vi "WPS_status.vi"() -> ()   [LabVIEW 2009]
panel:
  in  "Path to Exe":string="C:\\Documents and Settings\\Administrator\\My Documents\\LabViewProjects\\CTControl\\UU.W32.exe"
  out "error out":errorcluster
  out "outlet return":string
  out "Status Output":string
  in  "Password":string="WPS111rocks"
  in  "Username":string="admin"
  in  "WPS IP:Port":string="169.254.1.201:80"
  in  "Path to Batch":string="C:\\Documents and Settings\\Administrator\\My Documents\\LabViewProjects\\CTControl\\WPSrunExe.bat"
  in  "Outlet 8":bool
  in  "Outlet 7":bool
  in  "Outlet 6":bool
  in  "Outlet 5":bool
  in  "Outlet 4":bool
  in  "Outlet 3":bool
  in  "Outlet 2":bool
  in  "Outlet 1":bool
  in  "stop":bool
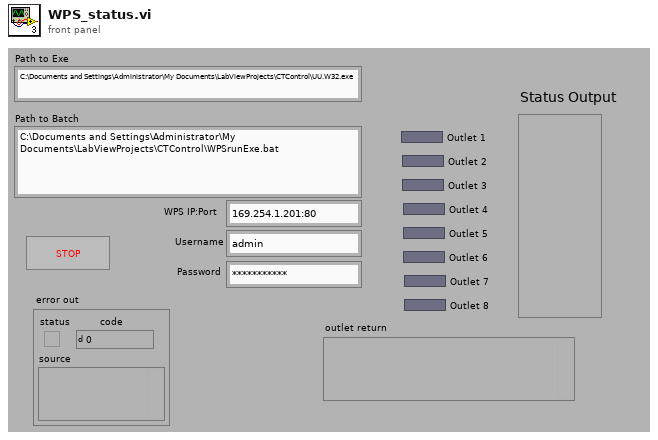
[diagram p1: front panel]
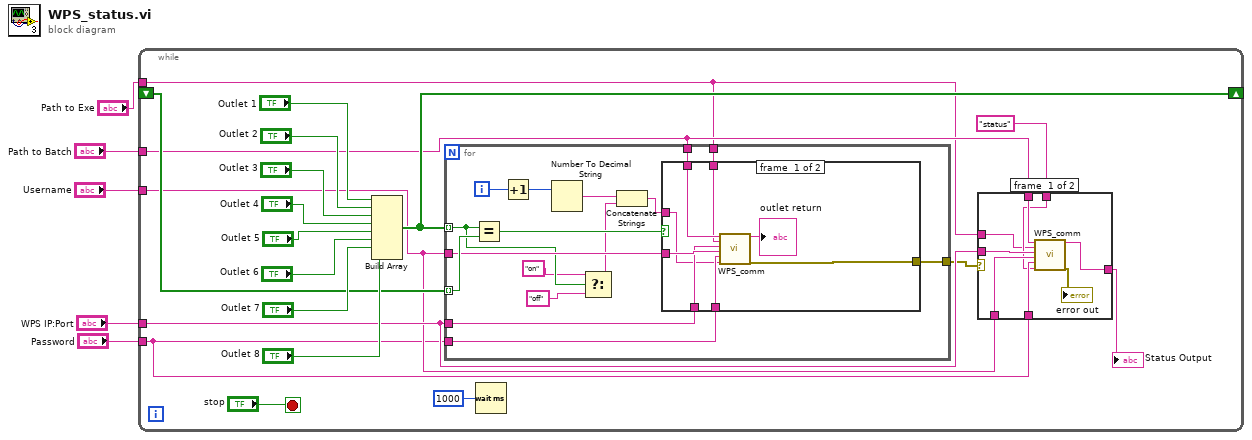
[diagram p0: block diagram]
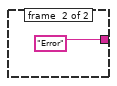
[diagram p2: hidden frame]
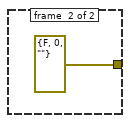
[diagram p3: hidden frame]
diagram:
  n1 = while {
    shift-right: [w16] -> _
    shift-left: _ -> [w15]
    tunnel: "Path to Batch" -> [w14]
    tunnel: "Username" -> [w12]
    tunnel: "WPS IP:Port" -> [w13]
    tunnel: "Password" -> [w11]
    tunnel: "Path to Exe" -> [w6]
    stop <- "stop" stop-if-true
    n2 = Build Array("Outlet 1", "Outlet 2", "Outlet 3", "Outlet 4", "Outlet 5", "Outlet 6", "Outlet 7", "Outlet 8") -> (w16:bool[])
    n3 = for {
      tunnel: w16 -> [w45] mode=indexing
      tunnel: w15 -> [w50] mode=indexing
      tunnel: w14 -> [w48]
      tunnel: w12 -> [w47]
      tunnel: w13 -> [w38]
      tunnel: w11 -> [w46]
      tunnel: [w39] -> w9
      tunnel: w6 -> [w35]
      i -> [w37]
      n4 = Equal?(x=w45, y=w50) -> (x = y?=w49:bool)
      n5 = Increment(x=w37) -> (x+1=w36:i32)
      n6 = Number To Decimal String(number=w36) -> (decimal integer string=w42:string)  [unwired: 1 in]
      n7 = Select(t="on", s=w45, f="off") -> (s? t:f=w41:string)
      n8 = Concatenate Strings(w42, w41) -> (w40:string)
      n9 = case shown="False" w49 {
        tunnel: w48 -> [w58 _]
        tunnel: w47 -> [w57 _]
        tunnel: w38 -> [w56 _]
        tunnel: w46 -> [w55 _]
        tunnel: w40 -> [w54 _]
        tunnel: [w53 errorcluster {"status"=FALSE, "code"=0, "source"=""} ("error out")] -> w39
        tunnel: w35 -> [w51 _]
        frame #0 {
          n10 = call "WPS_comm.vi"("Path to Batch"=w58, "Path to Exe"=w51, "WPS IP:Port"=w56, "Username"=w57, "Password"=w55, "Command"=w54) -> ("standard output"=→"outlet return":string, "error out"=w53:errorcluster)  [unwired: 10 in, 2 out]
        }
        frame #1 {
        }
      }
    }
    n11 = Wait (ms)(milliseconds to wait=u32 1000) -> ()  [unwired: 1 out]
    n12 = case shown="No Error" w9 {
      tunnel: w14 -> [w33 _]
      tunnel: w13 -> [w32 _]
      tunnel: w12 -> [w31 _]
      tunnel: w11 -> [w30 _]
      tunnel: "status" ("Command") -> [w27 _]
      tunnel: [w29 "Error"] -> w8
      tunnel: w6 -> [w26 _]
      frame #0 {
        n13 = call "WPS_comm.vi"("Path to Batch"=w33, "Path to Exe"=w26, "WPS IP:Port"=w32, "Username"=w31, "Password"=w30, "Command"=w27) -> ("standard output"=w29:string, "error out"=→"error out":errorcluster)  [unwired: 10 in, 2 out]
      }
      frame #1 {
      }
    }
    "Status Output" <- w8
  }
